vi "Post-BuildAction_CalcMD5_RTexe.vi"(5 "Files Generated by Build":path[](array[path]) caption="ビルドで生成されたファイル", 6 "Top Level/Always Included VIs":path[](array[path]) caption="トップレベル/常に含むVI", 7 "Destination Path":path caption="出力先パス", 8 "error in (no error)":errorcluster caption="エラー入力（エラーなし）", 9 "Target Name":string caption="ターゲット名", 10 "Build Specification Name":string caption="ビルド仕様名", 11 "Project Path":path caption="プロジェクトパス") -> (0 "error out":errorcluster caption="エラー出力")   [LabVIEW 2014]
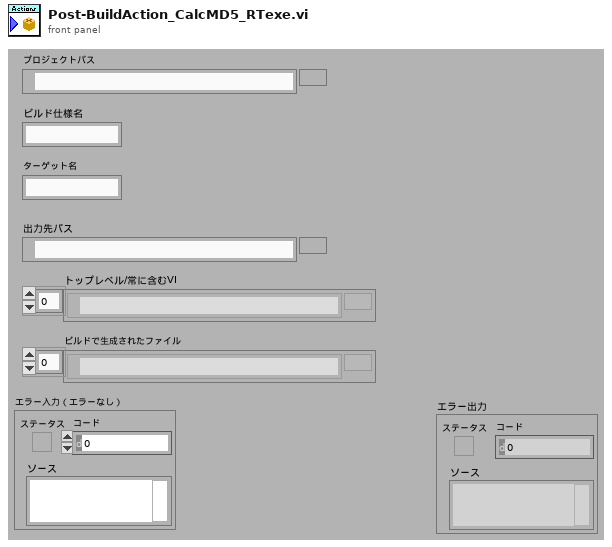
[diagram p1: front panel]
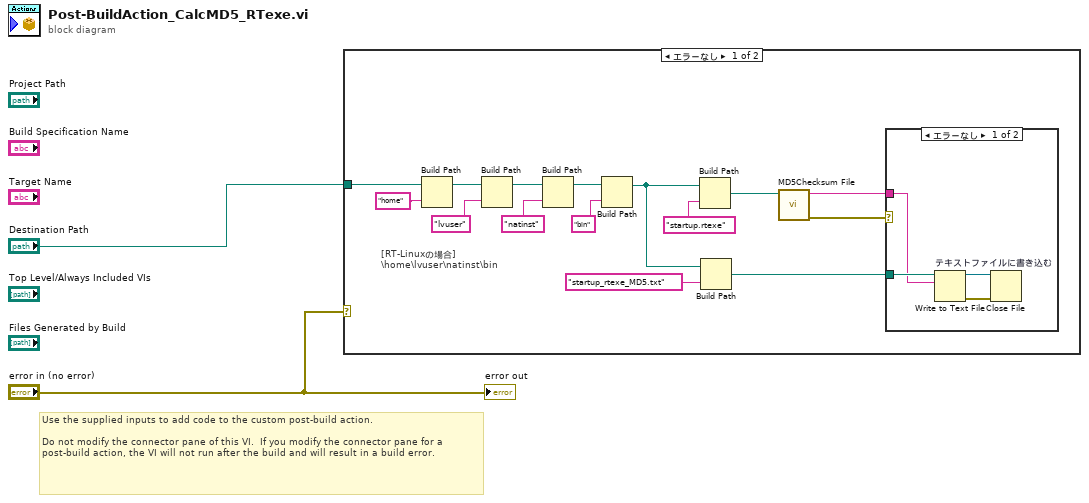
[diagram p0: block diagram]
diagram:
  # "Use the supplied inputs to add code to the custom post-build action.\n\nDo not modify the connector pane of this VI.  If you modify the connector pane for a post-build action, the VI will not run after the build and will result in a build error."
  n1 = case shown="エラーなし" "error in (no error)" {
    tunnel: "Destination Path" -> [w17 _]
    frame No Error {
      # "[RT-Linuxの場合]\n\\home\\lvuser\\natinst\\bin"
      n2 = Build Path(base path=w17, name or relative path="home" ("名前または相対パス")) -> (appended path=w15:path)
      n3 = Build Path(base path=w15, name or relative path="lvuser" ("名前または相対パス")) -> (appended path=w13:path)
      n4 = Build Path(base path=w13, name or relative path="natinst" ("名前または相対パス")) -> (appended path=w11:path)
      n5 = Build Path(base path=w11, name or relative path="bin" ("名前または相対パス")) -> (appended path=w7:path)
      n6 = Build Path(base path=w7, name or relative path="startup.rtexe" ("名前または相対パス")) -> (appended path=w8:path)
      n7 = Build Path(base path=w7, name or relative path="startup_rtexe_MD5.txt" ("名前または相対パス")) -> (appended path=w5:path)
      n8 = call <vilib>:"MD5Checksum File.vi"("Path"=w8) -> ("error out"=w6:errorcluster, "MD5 message-digest"=w3:string)  [unwired: 9 in]
      n9 = case shown="エラーなし" w6 {
        tunnel: w5 -> [w21 _]
        tunnel: w3 -> [w20 _]
        frame No Error {
          n10 = Write to Text File "テキストファイルに書き込む"(file (use dialog)=w21, text=w20) -> (refnum out=w19:refnum<file>, error out=w18:errorcluster)  [unwired: 2 in, 1 out]
          n11 = Close File(refnum=w19, error in=w18) -> ()  [unwired: 2 out]
        }
        frame Error {
        }
      }
    }
    frame Error {
    }
  }
  "error out" <- "error in (no error)"
